vi "Get View.vi"(8 "error in":errorcluster, 11 "Cell in":refnum<class "Cell.lvclass">) -> (0 "error out":errorcluster, 2 "View":refnum<class "Cell View.lvclass">, 3 "Cell out":refnum<class "Cell.lvclass">)   [LabVIEW 2024, in "SourceGrid.lvlib" / "Cell.lvclass"]
uses:
  Cell.lvclass
  Cell.lvclass/Cell.ctl
  D:/git/Sourcegrid-LabVIEW/dll/SourceGrid.dll
  dll/SourceGrid.dll
  Views/Cell View/Cell View.lvclass
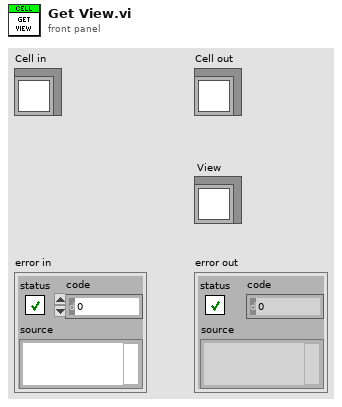
[diagram p1: front panel]
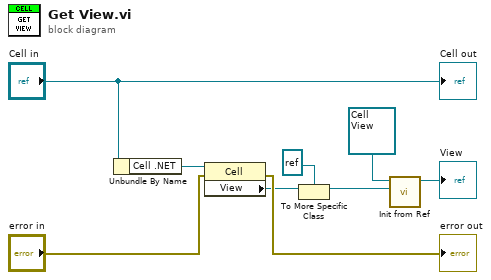
[diagram p0: block diagram]
diagram:
  n1 = Unbundle By Name("Cell in") -> ("Cell .NET"=w8:refnum<k24>)
  n2 = property class="Cell"(reference=w8, error in="error in") -> (error out=→"error out":errorcluster, "View"=w4:refnum<k24>)  [unwired: 1 out]
  n3 = To More Specific Class(target class=refnum<k24> refnum ("new reference"), reference=w4) -> (specific class reference=w2:refnum<k24>)  [unwired: 1 in, 1 out]
  n4 = call-dynamic "Init from Ref.vi"("Cell View .NET"=w2, "Cell View in"=refnum<class "Cell View.lvclass"> refnum) -> ("Cell View out"=→"View":refnum<class "Cell View.lvclass">)  [unwired: 9 in]
  "Cell out" <- "Cell in"
